vi "PalmSense Disconnect.vi"(8 "error in (no error)":errorcluster, 11 "Hardware Resources in":T1) -> (0 "error out":errorcluster, 3 "Hardware Resources out":T1)   [LabVIEW 2020, in "PalmSens.lvlib"]
doc: "Stops the acquisition."
uses:
  PalmSens.lvlib
  PalmSense Hardware Configuration.ctl
  <instrlib>/PalmSens SDK for LabVIEW 5.10/PalmSens/PalmSens.lvclass
  support/Message Queue/Message Cluster.ctl
  support/Message Queue/Message Queue.lvlib
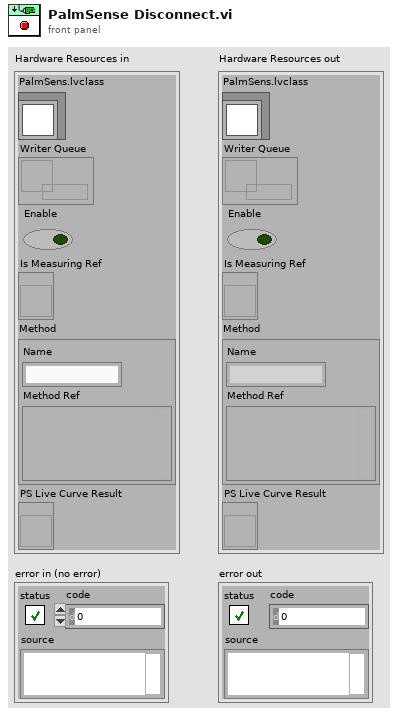
[diagram p1: front panel]
types:
  T1 = typedef "PalmSens.lvlib/PalmSense Hardware Configuration.ctl" = cluster{"PalmSens.lvclass":refnum<class "PalmSens.lvclass">, "Writer Queue":refnum<queue>, "Enable":bool, "Is Measuring Ref":refnum<vi>, "Method":cluster{"Name":string, "Method Ref":variant}, "PS Live Curve Result":refnum<vi>}
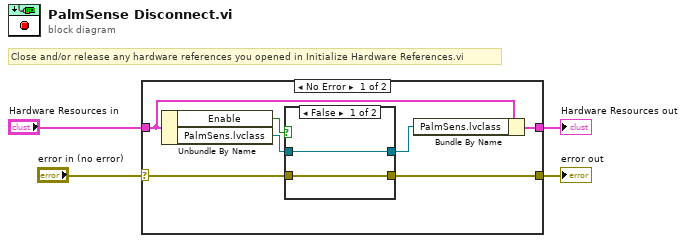
[diagram p0: block diagram]
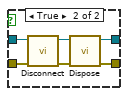
[diagram p2: hidden frame]
diagram:
  # "Close and/or release any hardware references you opened in Initialize Hardware References.vi"
  n1 = case shown="No Error" "error in (no error)" {
    selector: "error in (no error)" -> [w10 w21]
    tunnel: [w9 w21] -> w3
    tunnel: "Hardware Resources in" -> [w6 w20]
    tunnel: [w5 w20] -> w1
    frame No Error {
      n2 = Unbundle By Name(w6) -> ("Enable"=w8:bool, "PalmSens.lvclass"=w11:refnum<class "PalmSens.lvclass">)
      n3 = case shown="False" w8 {
        tunnel: w11 -> [w12 w19]
        tunnel: w10 -> [w13 w18]
        tunnel: [w13 w15] -> w9
        tunnel: [w12 w14] -> w7
        frame False {
        }
        frame True {
          n4 = call-dynamic "Disconnect.vi"("error in (no error)"=w18, "PalmSens in"=w19) -> ("error out"=w16:errorcluster, "PalmSens out"=w17:refnum<class "PalmSens.lvclass">)  [unwired: 8 in]
          n5 = call-dynamic "Dispose.vi"("error in (no error)"=w16, "PalmSens in"=w17) -> ("error out"=w15:errorcluster, "PalmSens out"=w14:refnum<class "PalmSens.lvclass">)  [unwired: 8 in]
        }
      }
      n6 = Bundle By Name(cluster=w6, "PalmSens.lvclass"=w7) -> (w5:T1)
    }
    frame Error {
    }
  }
  "error out" <- w3
  "Hardware Resources out" <- w1
